vi "Initialize.vi"(8 "error in (no error)":errorcluster, 11 "Panel Helper in":refnum<class "Panel Helper.lvclass">) -> (0 "error out":errorcluster, 2 "Created New?":bool, 3 "Panel Helper out":refnum<class "Panel Helper.lvclass">)   [LabVIEW 2019, in "Panel.lvlib" / "Panel Helper.lvclass"]
doc: "Makes sure the panel Helper is initialized. If not, it will create a new Panel Helper object.\n----\nCopyright: MGI 2017\nAuthor: Derek Trepanier"
uses:
  Panel Helper.lvclass
  Panel Helper.lvclass/Panel Helper.ctl
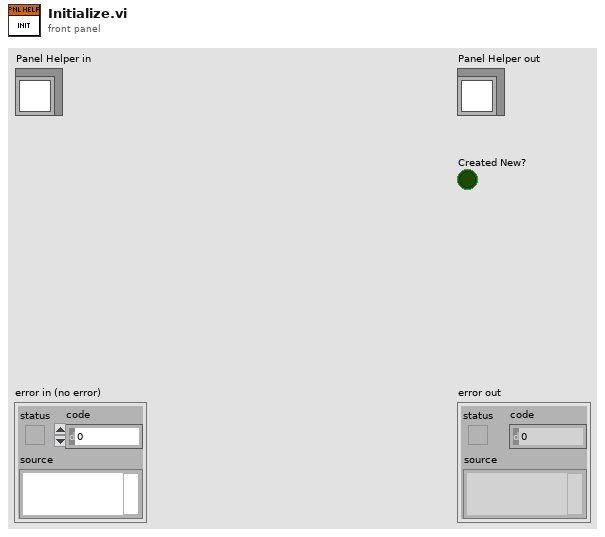
[diagram p1: front panel]
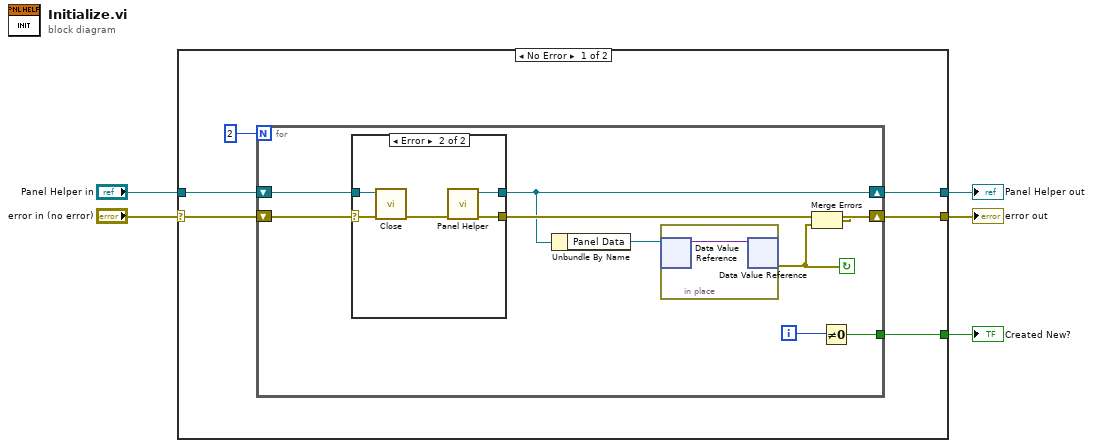
[diagram p0: block diagram]
diagram:
  n1 = case shown="No Error" "error in (no error)" {
    selector: "error in (no error)" -> [w8 w27]
    tunnel: [w8 w27] -> w4
    tunnel: [w6 w26] -> w2
    tunnel: "Panel Helper in" -> [w9 w26]
    tunnel: [w7 _] -> w1
    frame No Error {
      n2 = for {
        N: 2 -> [_]
        shift-right: [w17] -> w6
        shift-left: w9 -> [w19]
        shift-right: [w15] -> _
        shift-left: w8 -> [w18]
        tunnel: [w11] -> w7
        i -> [w12]
        stop <- w13 continue-if-true
        n3 = case shown="Error" w18 {
          selector: w18 -> [w20 _]
          tunnel: [w21 w24] -> w17
          tunnel: w19 -> [w21 w23]
          tunnel: [w20 w22] -> w16
          frame No Error {
          }
          frame Error {
            n4 = call "Close.vi"("Controller in"=w23) -> ()  [unwired: 10 in, 1 out]
            n5 = call "Panel Helper.vi"() -> ("Error Out"=w22:errorcluster, "Panel Helper out"=w24:refnum<class "Panel Helper.lvclass">)  [unwired: 9 in, 1 out]
          }
        }
        n6 = Unbundle By Name(w17) -> ("Panel Data"=w14:refnum<data-value>)
        n7 = in-place {
          n8 = in-place-dvr #1(w14) -> (w25:variant)  [unwired: 1 out]
          n9 = in-place-dvr #1(w25) -> (w13:errorcluster)  [unwired: 1 out]
        }
        n10 = Merge Errors(w16, w13) -> (w15:errorcluster)
        n11 = Not Equal To 0?(x=w12) -> (x != 0?=w11:bool)
      }
    }
    frame Error {
    }
  }
  "error out" <- w4
  "Panel Helper out" <- w2
  "Created New?" <- w1
